vi "SIM_Ion.vi"() -> (1 "Ion (ppm)":dbl format="%.2f")   [LabVIEW 2016]
panel:
  in  "sim_high":dbl=3000.0 format="%.2f"
  in  "sim_low":dbl=2900.0 format="%.2f"
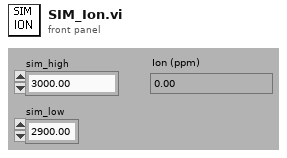
[diagram p1: front panel]
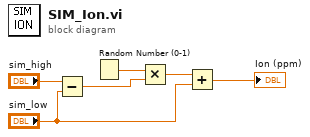
[diagram p0: block diagram]
diagram:
  n1 = Subtract(x="sim_high", y="sim_low") -> (x-y=w4:dbl)
  n2 = Random Number (0-1)() -> (number: 0 to 1=w5:dbl)
  n3 = Multiply(x=w5, y=w4) -> (x*y=w3:dbl)
  n4 = Add(x=w3, y="sim_low") -> (x+y=→"Ion (ppm)":dbl)
